vi "Impedance Equivalent Circuit Converter Vector.vi"(0 "major in":dbl[](array[numeric]), 1 "u(major) in":dbl[](array[numeric]), 2 "minor in":dbl[](array[numeric]), 3 "u(minor) in":dbl[](array[numeric]), 4 "f [Hz]":dbl[](array[numeric]), 5 "error in (no error)":errorcluster, 6 "type in":T2=enum."Rs-Xs", 7 "f scalar [Hz]":dbl, 8 "type in by string":string, 10 "type out by string":string, 12 "type out":T2=enum."Rs-Xs") -> (14 "major out":dbl[](array[numeric]), 15 "u(major) out":dbl[](array[numeric]), 16 "minor out":dbl[](array[numeric]), 17 "u(minor) out":dbl[](array[numeric]), 18 "type out info":T1, 19 "error out":errorcluster)   [LabVIEW 2020]
doc: "Impedance equivalent circuit connection converter. Identify input and output types either by type id or type string."
uses:
  Impedance Equivalent Circuit.ctl
  Impedance Equivalent Circuit Type Info.ctl
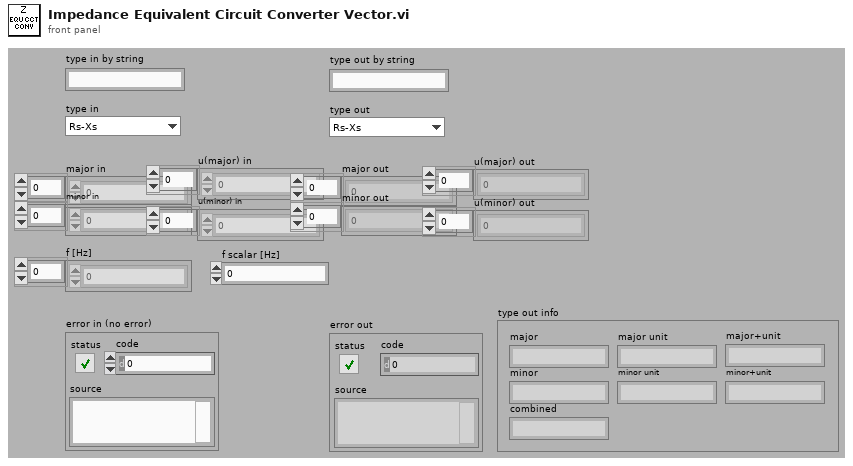
[diagram p1: front panel]
types:
  T1 = typedef "Impedance Equivalent Circuit Type Info.ctl" = cluster{"major":string, "major unit":string, "minor":string, "minor unit":string, "combined":string, "major+unit":string, "minor+unit":string}
  T2 = typedef "Impedance Equivalent Circuit.ctl" = enum16{"Keep original", "Rs-Xs", "Gp-Bp", "Z-phid", "Z-phir", "Y-phid", "Y-phir", "Cp-D", "Cp-Q", "Cp-Rp", "Cp-Gp", "Cs-D", "Cs-Q", "Cs-Rs", "Ls-Rs", "Ls-Q", "Rs-Tau", "Rp-Tau", "Lp-Q", "Lp-Rp"}
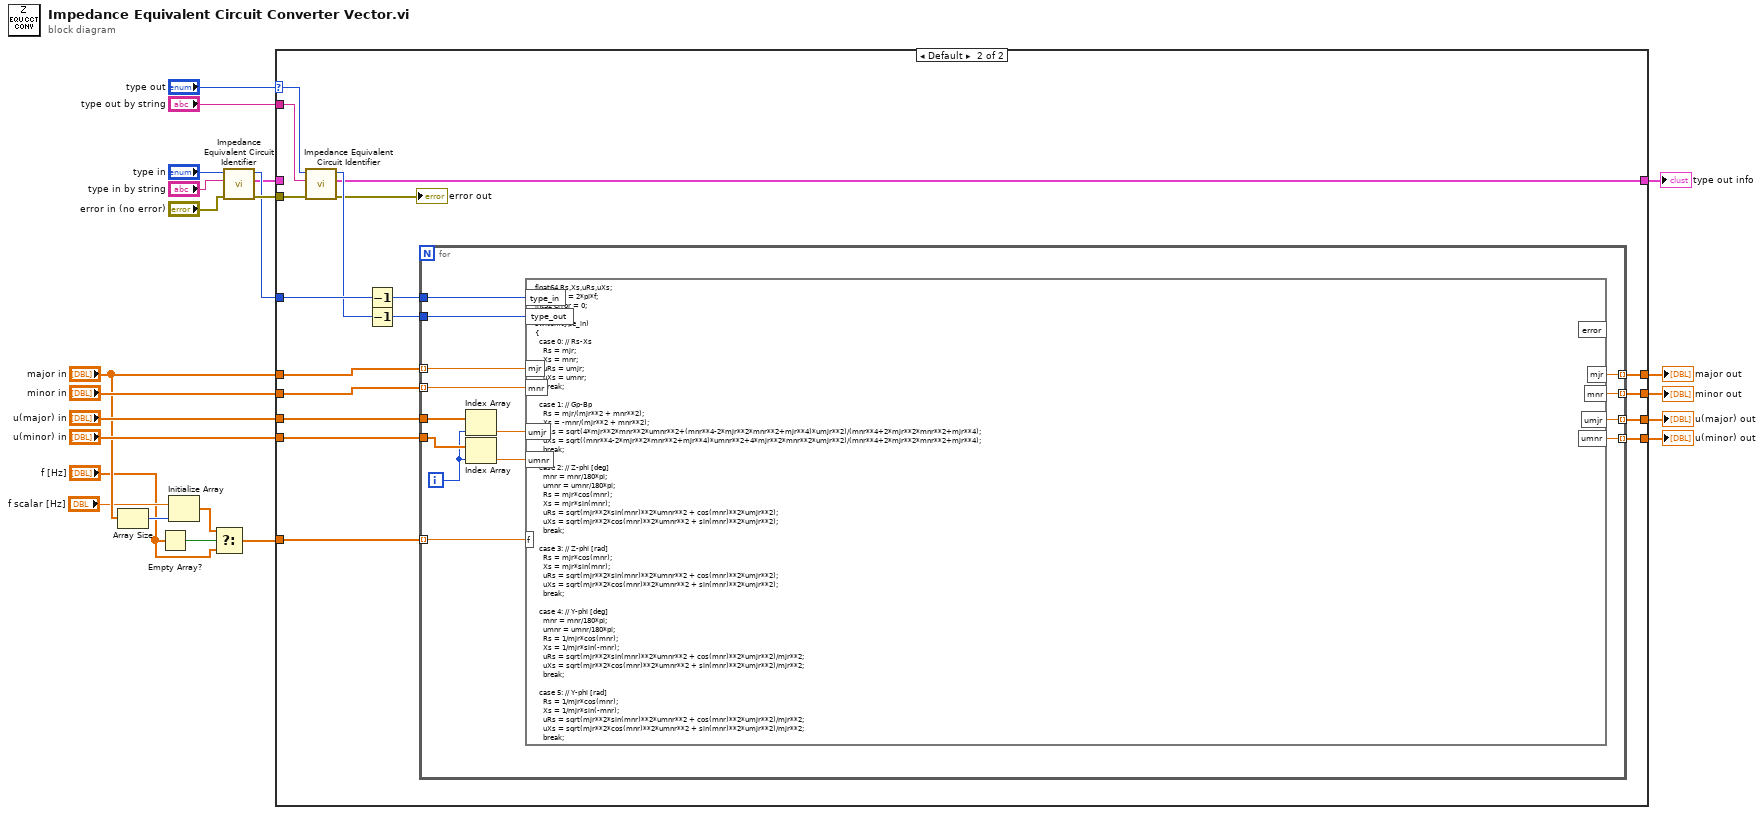
[diagram p0: block diagram]
diagram:
  n1 = Array Size(array="major in") -> (size(s)=w9:i32)
  n2 = Empty Array?(array="f [Hz]") -> (empty?=w10:bool)
  n3 = Initialize Array("f scalar [Hz]", w9) -> (w6:dbl[])
  n4 = Select(t=w6, s=w10, f="f [Hz]") -> (s? t:f=w4:dbl[])
  n5 = call "Impedance Equivalent Circuit Identifier.vi"("error in (no error)"="error in (no error)", "type in by string"="type in by string", "type in"="type in") -> ("error out"=w14:errorcluster, "type info"=w1:T1, "type out"=w12:T2)  [unwired: 6 in]
  n6 = case shown="Default" "type out" {
    selector: "type out" -> [_ w32]
    tunnel: "minor in" -> [w27 w46]
    tunnel: "u(major) in" -> [w26 w45]
    tunnel: "u(minor) in" -> [w25 w44]
    tunnel: [w28 w43] -> w20
    tunnel: [w27 w42] -> w19
    tunnel: [w26 w41] -> w18
    tunnel: [w25 w40] -> w17
    tunnel: w14 -> [_ w39]
    tunnel: "type out by string" -> [_ w38]
    tunnel: w12 -> [_ w37]
    tunnel: "major in" -> [w28 w34]
    tunnel: w4 -> [_ w33]
    tunnel: [w24 w31] -> w2
    tunnel: w1 -> [w24 _]
    frame "Keep original" {
    }
    frame Default {
      n7 = call "Impedance Equivalent Circuit Identifier.vi"("error in (no error)"=w39, "type in by string"=w38, "type in"=w32) -> ("error out"=→"error out":errorcluster, "type info"=w31:T1, "type out"=w36:T2)  [unwired: 6 in]
      n8 = Decrement(x=w37) -> (x-1=w30:T2)
      n9 = Decrement(x=w36) -> (x-1=w29:T2)
      n10 = for {
        tunnel: w29 -> [w60]
        tunnel: w34 -> [w59] mode=indexing
        tunnel: w46 -> [w58] mode=indexing
        tunnel: w45 -> [w51]
        tunnel: w44 -> [w48]
        tunnel: [w57] -> w43 mode=indexing
        tunnel: [w56] -> w42 mode=indexing
        tunnel: [w55] -> w41 mode=indexing
        tunnel: [w54] -> w40 mode=indexing
        tunnel: w30 -> [w53]
        tunnel: w33 -> [w52] mode=indexing
        i -> [w47]
        n11 = Index Array(array=w51, index=w47) -> (element=w50:dbl)
        n12 = Index Array(array=w48, index=w47) -> (element=w49:dbl)
        n13 = formula code="float64 Rs,Xs,uRs,uXs;\nfloat64 w = 2*pi*f;\nint32 error = 0;\n\nswitch(type_in)\n{\n  case 0: // Rs-Xs\n    Rs = mjr;\n    Xs = mnr;\n    uRs = umjr;\n    uXs = umnr;\n    break;\n\n  case 1: // Gp-Bp\n    Rs = mjr/(mjr**2 + mnr**2);\n    Xs = -mnr/(mjr**2 + mnr**2);                \n    uRs = sqrt(4*mjr**2*mnr**2*umnr**2+(mnr**4-2*mjr**2*mnr**2+mjr**4)*umjr**2)/(mnr**4+2*mjr**2*mnr**2+mjr**4);\n    uXs = sqrt((mnr**4-2*mjr**2*mnr**2+mjr**4)*umnr**2+4*mjr**2*mnr**2*umjr**2)/(mnr**4+2*mjr**2*mnr**2+mjr**4);\n    break;\n\n  case 2: // Z-phi [deg]\n    mnr = mnr/180*pi;\n    umnr = umnr/180*pi;\n    Rs = mjr*cos(mnr);\n    Xs = mjr*sin(mnr);\n    uRs = sqrt(mjr**2*sin(mnr)**2*umnr**2 + cos(mnr)**2*umjr**2);\n    uXs = sqrt(mjr**2*cos(mnr)**2*umnr**2 + sin(mnr)**2*umjr**2);\n    break;\n\n  case 3: // Z-phi [rad]\n    Rs = mjr*cos(mnr);\n    Xs = mjr*sin(mnr);\n    uRs = sqrt(mjr**2*sin(mnr)**2*umnr**2 + cos(mnr)**2*umjr**2);\n    uXs = sqrt(mjr**2*cos(mnr)**2*umnr**2 + sin(mnr)**2*umjr**2);        \n    break;\n  \n  case 4: // Y-phi [deg]\n    mnr = mnr/180*pi;\n    umnr = umnr/180*pi;\n    Rs = 1/mjr*cos(mnr);\n    Xs = 1/mjr*sin(-mnr);\n    uRs = sqrt(mjr**2*sin(mnr)**2*umnr**2 + cos(mnr)**2*umjr**2)/mjr**2;\n    uXs = sqrt(mjr**2*cos(mnr)**2*umnr**2 + sin(mnr)**2*umjr**2)/mjr**2;\n    break;\n                  \n  case 5: // Y-phi [rad]\n    Rs = 1/mjr*cos(mnr);\n    Xs = 1/mjr*sin(-mnr);\n    uRs = sqrt(mjr**2*sin(mnr)**2*umnr**2 + cos(mnr)**2*umjr**2)/mjr**2;\n    uXs = sqrt(mjr**2*cos(mnr)**2*umnr**2 + sin(mnr)**2*umjr**2)/mjr**2;\n    break;\n  \n  case 6: // Cp-D\n    Rs = mnr/((mjr*mnr**2+mjr)*w);\n    Xs = -1/((mjr*mnr**2+mjr)*w);\n    uRs = sqrt((mjr**2*mnr**4-2*mjr**2*mnr**2+mjr**2)*umnr**2+(mnr**6+2*mnr**4+mnr**2)*umjr**2)/((mjr**2*mnr**4+2*mjr**2*mnr**2+mjr**2)*abs(w));\n    uXs = sqrt(4*mjr**2*mnr**2*umnr**2+(mnr**4+2*mnr**2+1)*umjr**2)/((mjr**2*mnr**4+2*mjr**2*mnr**2+mjr**2)*abs(w));\n    break;\n                          \n  case 7: // Cp-Q\n    Rs = mnr/((mjr*mnr**2+mjr)*w);\n    Xs = -mnr**2/((mjr*mnr**2+mjr)*w);\n    uRs = sqrt((mjr**2*mnr**4-2*mjr**2*mnr**2+mjr**2)*umnr**2+(mnr**6+2*mnr**4+mnr**2)*umjr**2)/((mjr**2*mnr**4+2*mjr**2*mnr**2+mjr**2)*abs(w));\n    uXs = (mnr*sqrt(4*mjr**2*umnr**2+(mnr**6+2*mnr**4+mnr**2)*umjr**2))/((mjr**2*mnr**4+2*mjr**2*mnr**2+mjr**2)*abs(w));\n    break;\n          \n  case 8: // Cp-Rp\n    Rs = mnr/(mjr**2*mnr**2*w**2+1);\n    Xs = -(mjr*mnr**2*w)/(mjr**2*mnr**2*w**2+1);\n    uRs = sqrt((mjr**4*mnr**4*umnr**2+4*mjr**2*mnr**6*umjr**2)*w**4-2*mjr**2*mnr**2*umnr**2*w**2+umnr**2)/(mjr**4*mnr**4*w**4+2*mjr**2*mnr**2*w**2+1);\n    uXs = (mnr*w*sqrt(mjr**4*mnr**6*umjr**2*w**4-2*mjr**2*mnr**4*umjr**2*w**2+4*mjr**2*umnr**2+mnr**2*umjr**2))/(mjr**4*mnr**4*w**4+2*mjr**2*mnr**2*w**2+1); \n    break;\n          \n  case 9: // Cp-Gp\n    Rs = mnr/(mjr**2*w**2+mnr**2);\n    Xs = -(mjr*w)/(mjr**2*w**2+mnr**2);        \n    uRs = sqrt((mjr**4*umnr**2+4*mjr**2*mnr**2*umjr**2)*w**4-2*mjr**2*mnr**2*umnr**2*w**2+mnr**4*umnr**2)/(mjr**4*w**4+2*mjr**2*mnr**2*w**2+mnr**4);\n    uXs = (w*sqrt(mjr**4*umjr**2*w**4-2*mjr**2*mnr**2*umjr**2*w**2+4*mjr**2*mnr**2*umnr**2+mnr**4*umjr**2))/(mjr**4*w**4+2*mjr**2*mnr**2*w**2+mnr**4);\n    break;\n          \n  case 10: // Cs-D\n    Rs = mnr/(mjr*w);\n    Xs = -1/(mjr*w);\n    uRs = sqrt(mjr**2*umnr**2+mnr**2*umjr**2)/(mjr**2*abs(w));\n    uXs = abs(umjr)/(mjr**2*abs(w)); \n    break;\n          \n  case 11: // Cs-Q\n    Rs = 1/(mjr*mnr*w);\n    Xs = -1/(mjr*w);\n    uRs = sqrt(mjr**2*umnr**2+mnr**2*umjr**2)/(mjr**2*abs(w));\n    uXs = abs(umjr)/(mjr**2*abs(w)); \n    break;\n                \n  case 12: // Cs-Rs\n    Rs = mnr;\n    Xs = -1/(mjr*w);\n    uRs = abs(umnr);\n    uXs = abs(umjr)/(mjr**2*abs(w));\n    break;\n          \n  case 13: // Ls-Rs        \n    Rs = mnr;\n    Xs = mjr*w;\n    uRs = abs(umnr);\n    uXs = abs(umjr)*abs(w);\n    break;\n                  \n  case 14: // Ls-Q\n    Rs = mjr*w/mnr;\n    Xs = mjr*w;\n    uRs = (sqrt(mjr**2*umnr**2+mnr**2*umjr**2)*abs(w))/mnr**2;\n    uXs = abs(umjr)*abs(w);\n    break;\n          \n  case 15: // Rs-tau\n    Rs = mjr;\n    Xs = mjr*mnr*w;\n    uRs = abs(umjr);\n    uXs = (mjr**2*umnr**2+mnr**2*umjr**2)**0.5*abs(w);\n    break;\n\n  case 16: // Rp-tau\n    float64 Rp = mjr;\n    float64 tau = mnr;\n    float64 uRp = umjr;\n    float64 uTau = umnr;\n    Rs = Rp/(tau**2*w**2+1.0);\n    Xs = (Rp*tau*w)/(tau**2*w**2+1.0);\n    uRs = ((uRp/(tau**2*w**2+1))**2 + (uTau*(2*Rp*tau*w**2)/(tau**4*w**4+2*tau**2*w**2+1))**2)**0.5;\n    uXs = ((uRp*(tau*w)/(tau**2*w**2+1))**2 + (uTau*(Rp*tau**2*w**3-Rp*w)/(tau**4*w**4+2*tau**2*w**2+1))**2)**0.5;\n    break;\n\n  case 17: // Lp-Q\n    float64 Lp = mjr;\n    float64 Q = mnr;\n    float64 uLp = umjr;\n    float64 uQ = umnr;\n    Rs = (Lp*Q*w)/(Q**2+1);\n    Xs = (Lp*Q**2*w)/(Q**2+1);\n    uRs = ((uLp*(Q*w)/(Q**2+1))**2 + (uQ*((Lp*Q**2-Lp)*w)/(Q**4+2*Q**2+1))**2)**0.5;\n    uXs = ((uLp*(Q**2*w)/(Q**2+1))**2 + (uQ*(2*Lp*Q*w)/(Q**4+2*Q**2+1))**2)**0.5;\n    break;\n\n  case 18: // Lp-Rp\n  {\n    float64 Lp = mjr;\n    float64 Rp = mnr;\n    float64 uLp = umjr;\n    float64 uRp = umnr;\n    Rs = (Lp**2*Rp*w**2)/(Lp**2*w**2+Rp**2);\n    Xs = (Lp*Rp**2*w)/(Lp**2*w**2+Rp**2);\n    uRs = ((uLp*(2*Lp*Rp**3*w**2)/(Lp**4*w**4+2*Lp**2*Rp**2*w**2+Rp**4))**2 + (uRp*(Lp**4*w**4-Lp**2*Rp**2*w**2)/(Lp**4*w**4+2*Lp**2*Rp**2*w**2+Rp**4))**2)**0.5;\n    uXs = ((uLp*(Lp**2*Rp**2*w**3-Rp**4*w)/(Lp**4*w**4+2*Lp**2*Rp**2*w**2+Rp**4))**2 + (uRp*(2*Lp**3*Rp*w**3)/(Lp**4*w**4+2*Lp**2*Rp**2*w**2+Rp**4))**2)**0.5;\n    break;\n  }\n\n  default:\n    error = 1;\n}\n\n\nswitch(type_out)\n{\n  case 0: // Rs-Xs\n    mjr = Rs; \n    mnr = Xs;\n    umjr = abs(uRs);\n    umnr = abs(uXs);\n    break;\n  \n  case 1: // Gp-Bp\n    mjr = Rs/(Rs**2 + Xs**2);\n    mnr = -Xs/(Rs**2 + Xs**2);     \n    umjr = sqrt(4*Rs**2*Xs**2*uXs**2+(Xs**4-2*Rs**2*Xs**2+Rs**4)*uRs**2)/(Xs**4+2*Rs**2*Xs**2+Rs**4);\n    umnr = sqrt((Xs**4-2*Rs**2*Xs**2+Rs**4)*uXs**2+4*Rs**2*Xs**2*uRs**2)/(Xs**4+2*Rs**2*Xs**2+Rs**4);\n    break;\n                  \n  case 2: // Z-phi [deg]\n    mjr = (Rs**2 + Xs**2)**0.5;\n    mnr = atan2(Xs,Rs)*180/pi;\n    umjr = (Xs**2*uXs**2+Rs**2*uRs**2)**0.5/(Xs**2+Rs**2)**0.5;\n    umnr = (Rs**2*uXs**2+Xs**2*uRs**2)**0.5/(Xs**4+2*Rs**2*Xs**2+Rs**4)**0.5*180/pi;        \n    break;\n                  \n  case 3: // Z-phi [rad]\n    mjr = (Rs**2 + Xs**2)**0.5;\n    mnr = atan2(Xs,Rs);\n    umjr = (Xs**2*uXs**2+Rs**2*uRs**2)**0.5/(Xs**2+Rs**2)**0.5;\n    umnr = (Rs**2*uXs**2+Xs**2*uRs**2)**0.5/(Xs**4+2*Rs**2*Xs**2+Rs**4)**0.5;        \n    break;\n  \n  case 4: // Y-phi [deg]\n    mjr = (Rs**2 + Xs**2)**-0.5;\n    mnr = atan2(-Xs,Rs)*180/pi;\n    umjr = (Xs**2*uXs**2+Rs**2*uRs**2)**0.5/(Xs**6+3*Rs**2*Xs**4+3*Rs**4*Xs**2+Rs**6)**0.5;\n    umnr = (Rs**2*uXs**2+Xs**2*uRs**2)**0.5/(Xs**4+2*Rs**2*Xs**2+Rs**4)**0.5*180/pi;\n    break;\n                  \n  case 5: // Y-phi [rad]\n    mjr = (Rs**2 + Xs**2)**-0.5;\n    mnr = atan2(-Xs,Rs);\n    umjr = (Xs**2*uXs**2+Rs**2*uRs**2)**0.5/(Xs**6+3*Rs**2*Xs**4+3*Rs**4*Xs**2+Rs**6)**0.5;\n    umnr = (Rs**2*uXs**2+Xs**2*uRs**2)**0.5/(Xs**4+2*Rs**2*Xs**2+Rs**4)**0.5;\n    break;\n  \n  case 6: // Cp-D\n    mjr = -Xs/(Rs**2 + Xs**2)/w;\n    mnr = -Rs/Xs;\n    umjr = ((Xs**4-2*Rs**2*Xs**2+Rs**4)*uXs**2+4*Rs**2*Xs**2*uRs**2)**0.5/(w**2*Xs**8+4*Rs**2*w**2*Xs**6+6*Rs**4*w**2*Xs**4+4*Rs**6*w**2*Xs**2+Rs**8*w**2)**0.5;\n    umnr = (Rs**2*uXs**2+Xs**2*uRs**2)**0.5/abs(Xs)**2.0;\n    break;\n                  \n  case 7: // Cp-Q\n    mjr = -Xs/(Rs**2 + Xs**2)/w;\n    mnr = -Xs/Rs;\n    umjr = ((Xs**4-2*Rs**2*Xs**2+Rs**4)*uXs**2+4*Rs**2*Xs**2*uRs**2)**0.5/(w**2*Xs**8+4*Rs**2*w**2*Xs**6+6*Rs**4*w**2*Xs**4+4*Rs**6*w**2*Xs**2+Rs**8*w**2)**0.5;\n    umnr = (Rs**2*uXs**2+Xs**2*uRs**2)**0.5/abs(Rs)**2.0;\n    break;\n          \n  case 8: // Cp-Rp\n    mjr = -Xs/(Rs**2 + Xs**2)/w;\n    mnr = 1/(Rs/(Rs**2 + Xs**2));\n    umjr = ((Xs**4-2*Rs**2*Xs**2+Rs**4)*uXs**2+4*Rs**2*Xs**2*uRs**2)**0.5/(w**2*Xs**8+4*Rs**2*w**2*Xs**6+6*Rs**4*w**2*Xs**4+4*Rs**6*w**2*Xs**2+Rs**8*w**2)**0.5;\n    umnr = (4*Rs**2*Xs**2*uXs**2+(Xs**4-2*Rs**2*Xs**2+Rs**4)*uRs**2)**0.5/abs(Rs)**2.0; \n    break;\n          \n  case 9: // Cp-Gp\n    mjr = -Xs/(Rs**2 + Xs**2)/w;\n    mnr = Rs/(Rs**2 + Xs**2);\n    umjr = ((Xs**4-2*Rs**2*Xs**2+Rs**4)*uXs**2+4*Rs**2*Xs**2*uRs**2)**0.5/(w**2*Xs**8+4*Rs**2*w**2*Xs**6+6*Rs**4*w**2*Xs**4+4*Rs**6*w**2*Xs**2+Rs**8*w**2)**0.5;\n    umnr = (4*Rs**2*Xs**2*uXs**2+(Xs**4-2*Rs**2*Xs**2+Rs**4)*uRs**2)**0.5/(Xs**8+4*Rs**2*Xs**6+6*Rs**4*Xs**4+4*Rs**6*Xs**2+Rs**8)**0.5; \n    break;          \n\n  case 10: // Cs-D\n    mjr = -1/Xs/w;\n    mnr = -Rs/Xs;\n    umjr = abs(uXs)/(abs(w)**1.0*abs(Xs)**2.0);\n    umnr = (Rs**2*uXs**2+Xs**2*uRs**2)**0.5/abs(Xs)**2.0; \n    break;\n          \n  case 11: // Cs-Q\n    mjr = -1/Xs/w;\n    mnr = -Xs/Rs;\n    umjr = abs(uXs)/(abs(w)**1.0*abs(Xs)**2.0);\n    umnr = (Rs**2*uXs**2+Xs**2*uRs**2)**0.5/abs(Rs)**2.0; \n    break;\n                \n  case 12: // Cs-Rs\n    mjr = -1/Xs/w;\n    mnr = Rs;\n    umjr = abs(uXs)/(abs(w)**1.0*abs(Xs)**2.0);\n    umnr = abs(uRs); \n    break;\n          \n  case 13: // Ls-Rs\n    mjr = Xs/w;\n    mnr = Rs;\n    umjr = abs(uXs)/abs(w)**1.0;\n    umnr = abs(uRs); \n    break;\n                  \n  case 14: // Ls-Q\n    mjr = Xs/w;\n    mnr = Xs/Rs;\n    umjr = abs(uXs)/abs(w)**1.0;\n    umnr = (Rs**2*uXs**2+Xs**2*uRs**2)**0.5/abs(Rs)**2.0;\n    break;\n          \n  case 15: // Rs-tau\n    mjr = Rs;\n    mnr = Xs/(w*Rs);\n    umjr = abs(uRs);\n    umnr = (Rs**2*uXs**2+Xs**2*uRs**2)**0.5/(abs(Rs)**2.0*abs(w));\n    break;\n\n  case 16: // Rp-tau\n    mjr = (Xs**2+Rs**2)/Rs;\n    mnr = Xs/(Rs*w);\n    umjr = ((uRs*(Xs**2-Rs**2)/Rs**2)**2 + (uXs*(2*Xs)/Rs)**2)**0.5;\n    umnr = ((uRs*Xs/(Rs**2*w))**2 + (uXs*1/(Rs*w))**2)**0.5;\n    break;\n\n  case 17: // Lp-Q\n    mjr = (Xs**2+Rs**2)/(Xs*w);\n    mnr = Xs/Rs;\n    umjr = ((uRs*(2*Rs)/(Xs*w))**2 + (uXs*(Xs**2-Rs**2)/(Xs**2*w))**2)**0.5;\n    umnr = ((uRs*Xs/Rs**2)**2 + (uXs*1/Rs)**2)**0.5;\n    break;\n\n  case 18: // Lp-Rp\n    mjr = (Xs**2+Rs**2)/(Xs*w);\n    mnr = (Xs**2+Rs**2)/Rs;\n    umjr = ((uRs*(2*Rs)/(Xs*w))**2 + (uXs*(Xs**2-Rs**2)/(Xs**2*w))**2)**0.5;\n    umnr = ((uRs*(Xs**2-Rs**2)/Rs**2)**2 + (uXs*(2*Xs)/Rs)**2)**0.5;\n    break;\n\n  default:\n    error = 1;\n}"("type_in"=w53, "type_out"=w60, "mjr"=w59, "mnr"=w58, "umjr"=w50, "umnr"=w49, "f"=w52) -> ("mjr"=w57:dbl, "mnr"=w56:dbl, "umjr"=w55:dbl, "umnr"=w54:dbl)  [unwired: 1 out]
      }
    }
  }
  "major out" <- w20
  "u(major) out" <- w18
  "minor out" <- w19
  "u(minor) out" <- w17
  "type out info" <- w2
